vi "GetID.vi"() -> (2 "设置ID":string)   [LabVIEW 2013]
uses:
  GlobalValue.vi
  <vilib>/Utility/config.llb/Read Key (U32).vi
  <vilib>/Utility/config.llb/Write Key (U32).vi
  <vilib>/Utility/config.llb/NI_LVConfig.lvlib
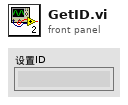
[diagram p1: front panel]
types:
  T1 = typedef "NI_LVConfig.lvlib/Config Data RefNum.ctl" = refnum<k1>
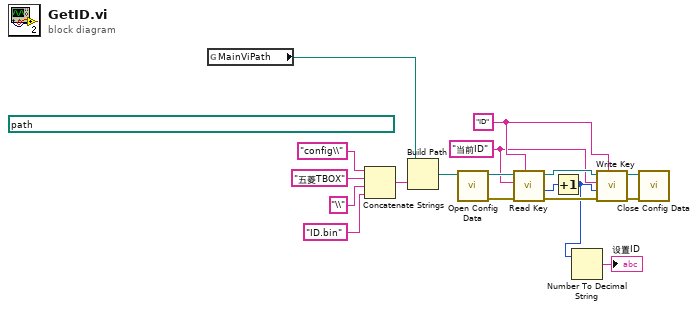
[diagram p0: block diagram]
diagram:
  w9 = "当前ID" ("key")
  w10 = "ID" ("section")
  (unwired) path "D:/赛格/T-BOX/T-BOX TestSystem/SourceCode/五菱T-BOX TestSystem" ("基路径")
  n1 = global read "GlobalValue.vi" "MainViPath"() -> (w1:path)
  n2 = Concatenate Strings("config\\" ("连接的字符串"), "五菱TBOX" ("字符串"), "\\" ("字符串"), "ID.bin" ("连接的字符串")) -> (w15:string)
  n3 = Build Path(base path=w1, name or relative path=w15) -> (appended path=w5:path)
  n4 = call <vilib>:"Open Config Data.vi"("configuration file path"=w5) -> ("error out"=w6:errorcluster, "refnum"=w13:T1)  [unwired: 8 in, 1 out]
  n5 = call-poly <vilib>:"Read Key.vi"("section"=w10, "error in (no error)"=w6, "key"=w9, "refnum"=w13) -> ("error out"=w7:errorcluster, "value"=w4:u32, "refnum out"=w12:T1)  [unwired: 4 in, 1 out]
  n6 = Increment(x=w4) -> (x+1=w2:u32)
  n7 = Number To Decimal String(number=w2) -> (decimal integer string=→"设置ID":string)  [unwired: 1 in]
  n8 = call-poly <vilib>:"Write Key.vi"("section"=w10, "error in (no error)"=w7, "value"=w2, "key"=w9, "refnum"=w12) -> ("error out"=w8:errorcluster, "refnum out"=w11:T1)  [unwired: 4 in, 1 out]
  n9 = call <vilib>:"Close Config Data.vi"("error in (no error)"=w8, "refnum"=w11) -> ()  [unwired: 8 in, 2 out]
